vi "Exercises_4-7.vi"() -> ()   [LabVIEW 2014]
panel:
  out "Square Root":dbl
  in  "Number":dbl
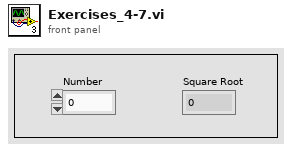
[diagram p1: front panel]
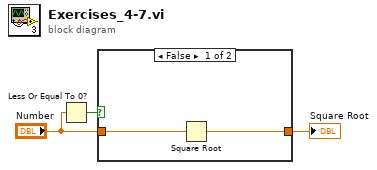
[diagram p0: block diagram]
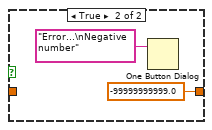
[diagram p2: hidden frame]
diagram:
  n1 = Less Or Equal To 0?(x="Number") -> (x <= 0?=w3:bool)
  n2 = case shown="False" w3 {
    tunnel: [w4 -99999999999.0] -> w1
    tunnel: "Number" -> [w5 _]
    frame False {
      n3 = Square Root(x=w5) -> (sqrt(x)=w4:dbl)
    }
    frame True {
      n4 = One Button Dialog(message="Error...\nNegative number") -> ()  [unwired: 1 in, 1 out]
    }
  }
  "Square Root" <- w1
